vi "ToteDrive.vi"(10 "Speed":dbl) -> (2 "Done?":bool)   [LabVIEW 2014]
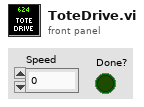
[diagram p1: front panel]
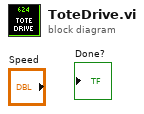
[diagram p0: block diagram]
diagram:
